vi "FlpLib SpaceVectorPWM 0.vi"(0 "ref_alpha":sgl caption="voltage alpha", 1 "ref_max":sgl=0.9999695, 2 "Period":i32=1, 5 "ref_beta":sgl caption="voltage beta") -> (4 "A":T1, 6 "B":T1, 8 "C":T1, 15 "Sector":u8)   [LabVIEW 2017]
uses:
  ON_OFF.ctl
  <userlib>/_NI FLP Library/FPGA/outsideSCTL/FlpLib Divide Shared Instance 0.vi
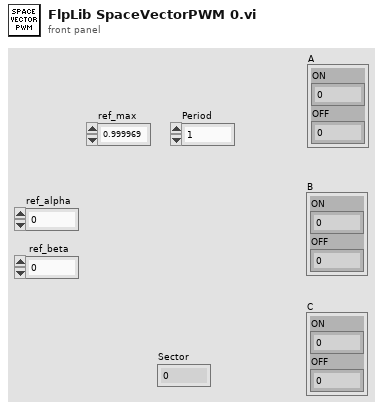
[diagram p1: front panel]
types:
  T1 = typedef "ON_OFF.ctl" = cluster{"ON":u32, "OFF":u32}
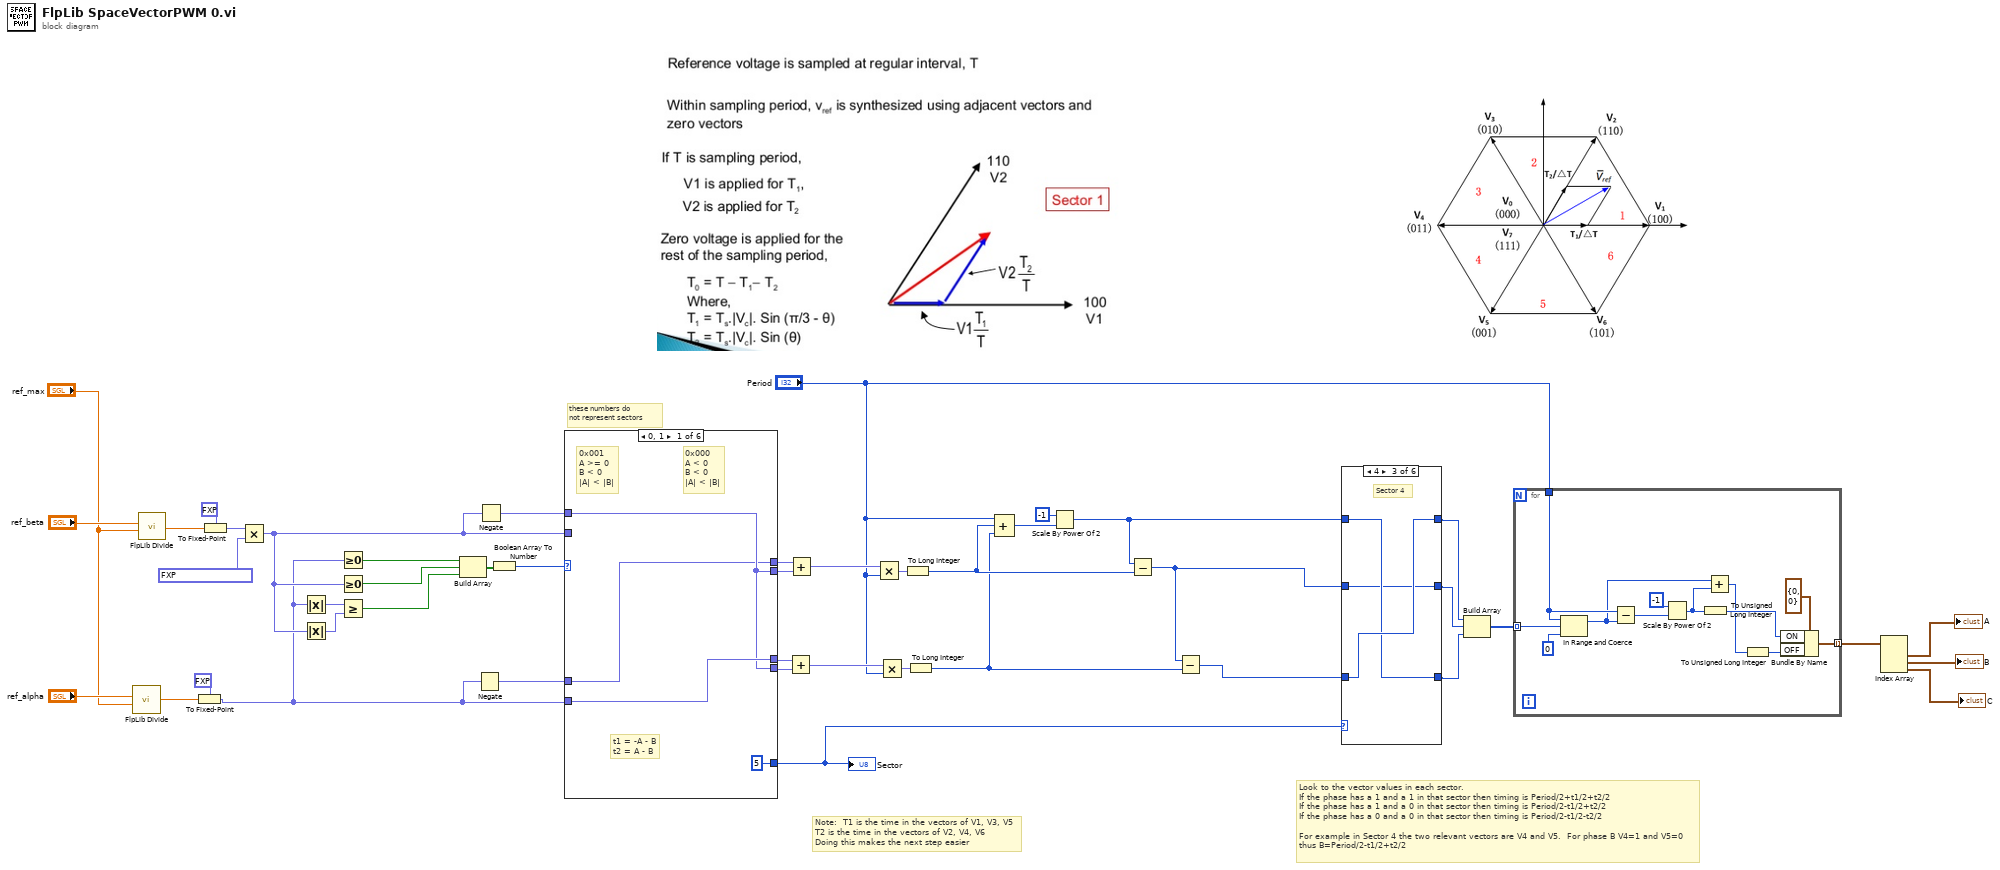
[diagram p0: block diagram]
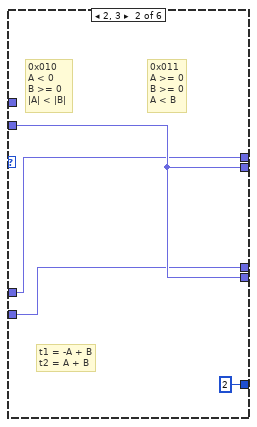
[diagram p7: hidden frame]
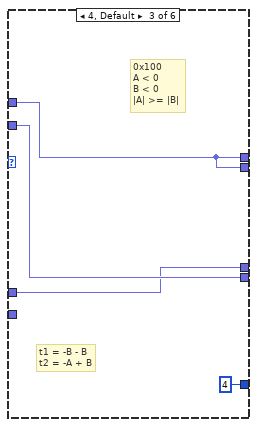
[diagram p8: hidden frame]
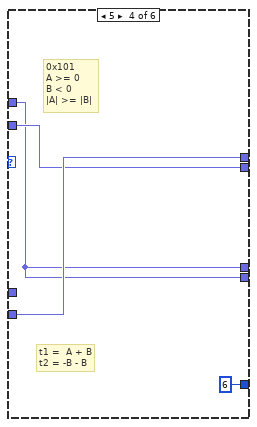
[diagram p9: hidden frame]
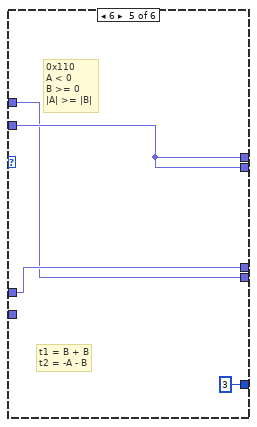
[diagram p10: hidden frame]
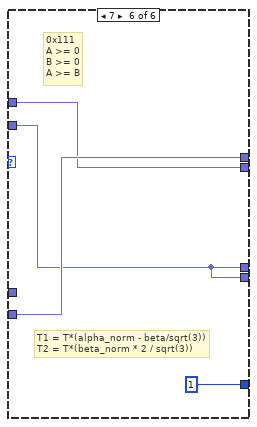
[diagram p11: hidden frame]
diagram:
  # "Note:  T1 is the time in the vectors of V1, V3, V5\nT2 is the time in the vectors of V2, V4, V6\nDoing this makes the next step easier"
  # "Look to the vector values in each sector.\nIf the phase has a 1 and a 1 in that sector then timing is Period/2+t1/2+t2/2\nIf the phase has a 1 and a 0 in that sector then timing is Period/2-t1/2+t2/2\nIf the phase has a 0 and a 0 in that sector then timing is Period/2-t1/2-t2/2\n\nFor example in Sector 4 the two relevant vectors are V4 and V5.  For phase B V4=1 and V5=0\nthus B=Period/2-t1/2+t2/2"
  # "these numbers do \nnot represent sectors"
  n1 = call-poly <userlib>:"FlpLib Divide.vi"("y"="ref_max", "x"="ref_alpha") -> ("x/y"=w5:sgl)  [unwired: 5 in]
  n2 = call-poly <userlib>:"FlpLib Divide.vi"("y"="ref_max", "x"="ref_beta") -> ("x/y"=w9:sgl)  [unwired: 5 in]
  n3 = To Fixed-Point(fixed-point type=fxp<+/-,24,2> 0.0, number=w5) -> (fixed-point=w4:fxp<+/-,24,2>)
  n4 = To Fixed-Point(fixed-point type=fxp<+/-,18,2> 0.0, number=w9) -> (fixed-point=w8:fxp<+/-,18,2>)
  n5 = Multiply(x=w8, y=fxp<+/-,18,2> 0.577362060546875 ("fixed-point type")) -> (x*y=w35:fxp<+/-,24,2>)
  n6 = Absolute Value(x=w4) -> (abs(x)=w41:fxp<+,24,2>)
  n7 = Absolute Value(x=w35) -> (abs(x)=w40:fxp<+,24,2>)
  n8 = Greater Or Equal To 0?(x=w4) -> (x >= 0?=w38:bool)
  n9 = Greater Or Equal To 0?(x=w35) -> (x >= 0?=w37:bool)
  n10 = Greater Or Equal?(x=w41, y=w40) -> (x >= y?=w36:bool)
  n11 = Build Array(w38, w37, w36) -> (w39:bool[])
  n12 = Negate(x=w4) -> (-x=w33:fxp<+/-,25,3>)
  n13 = Negate(x=w35) -> (-x=w34:fxp<+/-,25,3>)
  n14 = Boolean Array To Number(Boolean array=w39) -> (number=w25:u8)
  n15 = case shown="0, 1" w25 {
    tunnel: w35 -> [_ w53 w57 w60 w65 w68]
    tunnel: w4 -> [w49 w52 _ w61 _ w69]
    tunnel: [w47 w51 w56 w61 w65 w69] -> w45
    tunnel: [w48 w53 w56 w60 w65 w67] -> w44
    tunnel: [w49 w52 w55 w59 w64 w68] -> w43
    tunnel: [w48 w53 w57 w59 w63 w68] -> w42
    tunnel: w34 -> [w48 _ w56 w59 w63 w67]
    tunnel: w33 -> [w47 w51 w55 _ w64 _]
    tunnel: [u8 5 u8 2 u8 4 u8 6 u8 3 u8 1] -> w24
    frame 0, 1 {
      # "0x000\nA < 0\nB < 0\n|A| < |B|"
      # "t1 = -A - B\nt2 = A - B"
      # "0x001\nA >= 0\nB < 0\n|A| < |B|"
    }
    frame 2, 3 {
      # "0x011\nA >= 0\nB >= 0\nA < B"
      # "t1 = -A + B\nt2 = A + B"
      # "0x010\nA < 0\nB >= 0\n|A| < |B|"
    }
    frame 4, Default {
      # "t1 = -B - B\nt2 = -A + B"
      # "0x100\nA < 0\nB < 0\n|A| >= |B|"
    }
    frame 5 {
      # "t1 =  A + B\nt2 = -B - B"
      # "0x101\nA >= 0\nB < 0\n|A| >= |B|"
    }
    frame 6 {
      # "t1 = B + B\nt2 = -A - B"
      # "0x110\nA < 0\nB >= 0\n|A| >= |B|"
    }
    frame 7 {
      # "T1 = T*(alpha_norm - beta/sqrt(3))\nT2 = T*(beta_norm * 2 / sqrt(3))"
      # "0x111\nA >= 0\nB >= 0\nA >= B"
    }
  }
  "Sector" <- w24
  n16 = Add(x=w43, y=w42) -> (x+y=w28:fxp<+/-,26,4>)
  n17 = Add(x=w45, y=w44) -> (x+y=w29:fxp<+/-,26,4>)
  n18 = Multiply(x=w29, y="Period") -> (x*y=w17:fxp<+/-,57,35>)
  n19 = Multiply(x=w28, y="Period") -> (x*y=w16:fxp<+/-,57,35>)
  n20 = To Long Integer(number=w17) -> (32bit integer=w11:i32)
  n21 = To Long Integer(number=w16) -> (32bit integer=w10:i32)
  n22 = Compound Arithmetic op=ADD("Period", w11, w10) -> (w27:i32)
  n23 = Scale By Power Of 2(n=i16 -1, x=w27) -> (x*2^n=w13:i32)
  n24 = Subtract(x=w13, y=w11) -> (x-y=w15:i32)
  n25 = Subtract(x=w15, y=w10) -> (x-y=w14:i32)
  n26 = case shown="4" w24 {
    tunnel: w15 -> [w72 w75 w76 w79 w82 w86]
    tunnel: w13 -> [w71 w74 w77 w81 w83 w87]
    tunnel: w14 -> [w70 w73 w78 w80 w84 w85]
    tunnel: [w71 w73 w77 w79 w82 w85] -> w21
    tunnel: [w70 w74 w76 w80 w83 w86] -> w22
    tunnel: [w72 w75 w78 w81 w84 w87] -> w23
    frame 5 {
      # "Sector 5"
    }
    frame 2 {
      # "Sector 2"
    }
    frame 4 {
      # "Sector 4"
    }
    frame 6 {
      # "Sector 6"
    }
    frame 3 {
      # "sector 3"
    }
    frame 1, Default {
      # "Sector 1"
    }
  }
  n27 = Build Array(w23, w22, w21) -> (w20:i32[])
  n28 = for {
    tunnel: w20 -> [w99] mode=indexing
    tunnel: "Period" -> [w96]
    tunnel: [w94] -> w19 mode=indexing
    n29 = In Range and Coerce(upper limit=w96, x=w99, lower limit=0) -> (coerced(x)=w95:i32)  [unwired: 1 out]
    n30 = Subtract(x=w96, y=w95) -> (x-y=w97:i32)
    n31 = Scale By Power Of 2(n=i16 -1, x=w97) -> (x*2^n=w92:i32)
    n32 = To Unsigned Long Integer(number=w92) -> (unsigned 32bit integer=w91:u32)
    n33 = Add(x=w95, y=w92) -> (x+y=w89:i32)
    n34 = To Unsigned Long Integer(number=w89) -> (unsigned 32bit integer=w90:u32)
    n35 = Bundle By Name(cluster=T1 {"ON"=0, "OFF"=0} ("A"), "ON"=w91, "OFF"=w90) -> (w94:T1)
  }
  n36 = Index Array(array=w19) -> (element #1=→"A":T1, element #2=→"B":T1, element #3=→"C":T1)  [unwired: 3 in]
